vi "PID control.vi"() -> ()   [LabVIEW 2017]
uses:
  <vilib>/Simulation/Scripting/Companion Diagram/SimConfigNode/SimParams.ctl
  <vilib>/Simulation/Scripting/Companion Diagram/SimConfigNode/_simSolvers.ctl
  <vilib>/Simulation/Implementation/Shared/SIMSCR Execution Mode.ctl
  <vilib>/Simulation/Param Hierarchy/Typedefs/SIMPH Param Control Actions.ctl
  <vilib>/Simulation/Implementation/Shared/NILVSim_ParamChanged.vi
  <vilib>/Simulation/Implementation/Shared/NILVSIM_BeginStep.vi
  <vilib>/Simulation/Implementation/Shared/NILVSim_Manager.vi
  <vilib>/Utility/error.llb/Clear Errors.vi
  <vilib>/Simulation/Implementation/Shared/NILVSim_FinalizeModel.vi
  <vilib>/DAQmx/read.llb/DAQmx Read (Counter DBL 1Chan 1Samp).vi
  <vilib>/DAQmx/read.llb/DAQmx Read (Digital Bool 1Line 1Point).vi
  917b7e52-755f-4d44-bea8-9e7c9beac24e.vi
  a58f9967-76f1-4ebc-ad3d-26e75a3ca160.vi
  <vilib>/DAQmx/write.llb/DAQmx Write (Analog DBL 1Chan 1Samp).vi
  <vilib>/DAQmx/create/channels.llb/DAQmx Create Channel (AO-Voltage-Basic).vi
  <vilib>/DAQmx/create/channels.llb/DAQmx Create Channel (DI-Digital Input).vi
  <vilib>/DAQmx/create/channels.llb/DAQmx Create Channel (CI-Count Edges).vi
  <vilib>/Simulation/Implementation/Shared/SIM Unbundle Sim Info.vi
  <vilib>/Simulation/Implementation/Shared/NILVSim_Initialize.vi
  <vilib>/Simulation/Utility/Implementation/NILVSim Get Time and IsAcceptedStep.vi
  <vilib>/Simulation/Implementation/Shared/SIMSH Read Queue.vi
  <vilib>/Simulation/Implementation/Shared/NILVSim_GetModelError.vi
  <vilib>/Simulation/Implementation/Shared/SIM Bundle Sim Info.vi
  <vilib>/DAQmx/miscellaneous.llb/DAQmx Fill In Error Info.vi
  <vilib>/Simulation/Implementation/XNodeFramework/SimXNode/SimX.xnode
  <vilib>/Simulation/Model Libraries/PID/SIM PID (Parallel).vi
  <vilib>/Simulation/Model Libraries/PID/SIM PID.vi
  <vilib>/Simulation/Scripting/Companion Diagram/SimConfigNode/SimDog.xnode
  <vilib>/Simulation/Model Libraries/PID/SIM PID (Academic).vi
  <vilib>/Simulation/Implementation/Shared/NI_SIM_Implementation.lvlib
panel:
  out "x circle":bool
  out "y circle":bool
  out "Point circle is drawing":dbl
  out "false":bool
  in  "Radius 2":dbl
  out "No of Points":dbl
  out "Numeric y 2":dbl
  out "Y array 2":dbl[](array[numeric])
  out "array Y length 2":dbl
  out "Numeric x 2":dbl
  out "X array 2":dbl[](array[numeric])
  out "array x Length 2":dbl
  in  "stage circle":T1(ring)
  in  "check instruc":bool
  out "down 2":bool
  out "down":bool
  out "right":bool
  out "x entered":dbl
  out "y enetred":dbl
  out "greater -1 x":bool
  out "less 1 x":bool
  out "direction selected":dbl
  out "circle reset":bool
  in  "part circle":T2(ring)=enum."a"
  out "at 2f":bool
  out "Step 2J":bool
  out "Step 2H":bool
  out "Shape drawing steps":enum16{"corner", "1st switch", "reverse"}(ring)
  out "Step 2D":bool
  out "Step 2C":bool
  out "c":bool
  in  "height":dbl
  in  "length":dbl
  in  "part":T3(ring)=enum."a"
  out "Step 2A":bool
  out "Step 2B":bool
  in  "Has encoders been reset?":enum16{"don't reset", "reset"}(ring)
  out "x distance currently being travelled":dbl
  out "y distance currently being travelled":dbl
  out "error calced":dbl
  out "p1 dis 2":dbl
  out "p1 dis":dbl
  out "error y":dbl
  out "calc distance y":dbl
  out "calc distanc x":dbl
  out "error x":dbl
  out "reached y":bool
  out "reached x":bool
  out "Numeric":dbl
  in  "Draw rectangle":bool
  in  "Draw circle":bool
  out "In drawing mode":bool
  in  "Right-Down":bool
  in  "Left-Up":bool
  in  "Left-Down":bool
  in  "Right-Up":bool
  in  "right":bool
  in  "left":bool
  in  "motor 2":dbl(slide)=1.5 scale=-10.0..10.0
  in  "down":bool
  in  "up":bool
  in  "Y Length":dbl=30.0
  in  "X Length":dbl=30.0
  in  "Motor 2 encoder":tag="Dev1/ctr1"
  out "Pulses M2":dbl format="%.2f"
  in  "Motor 1 encoder":tag="Dev1/ctr0"
  out "Pulses M1":dbl format="%.2f"
  out "Right":bool
  out "Bottom":bool
  out "Left":bool
  out "Top":bool
  in  "Switch 4/Line 3":tag="Dev1/port0/line3"
  in  "Switch 3/Line 2":tag="Dev1/port0/line2"
  in  "Switch 2/Line 1":tag="Dev1/port0/line1"
  in  "Switch 1/Line 0":tag="Dev1/port0/line0"
  in  "Motor stop":bool
  in  "Motor 1":tag="Dev1/ao0"
  in  "max Voltage":dbl=10.0
  in  "Min Voltage":dbl=-10.0
  in  "Motor 2":tag="Dev1/ao1"
  in  "motor 1":dbl(slide)=1.5 scale=-10.0..10.0
  in  "stop":bool
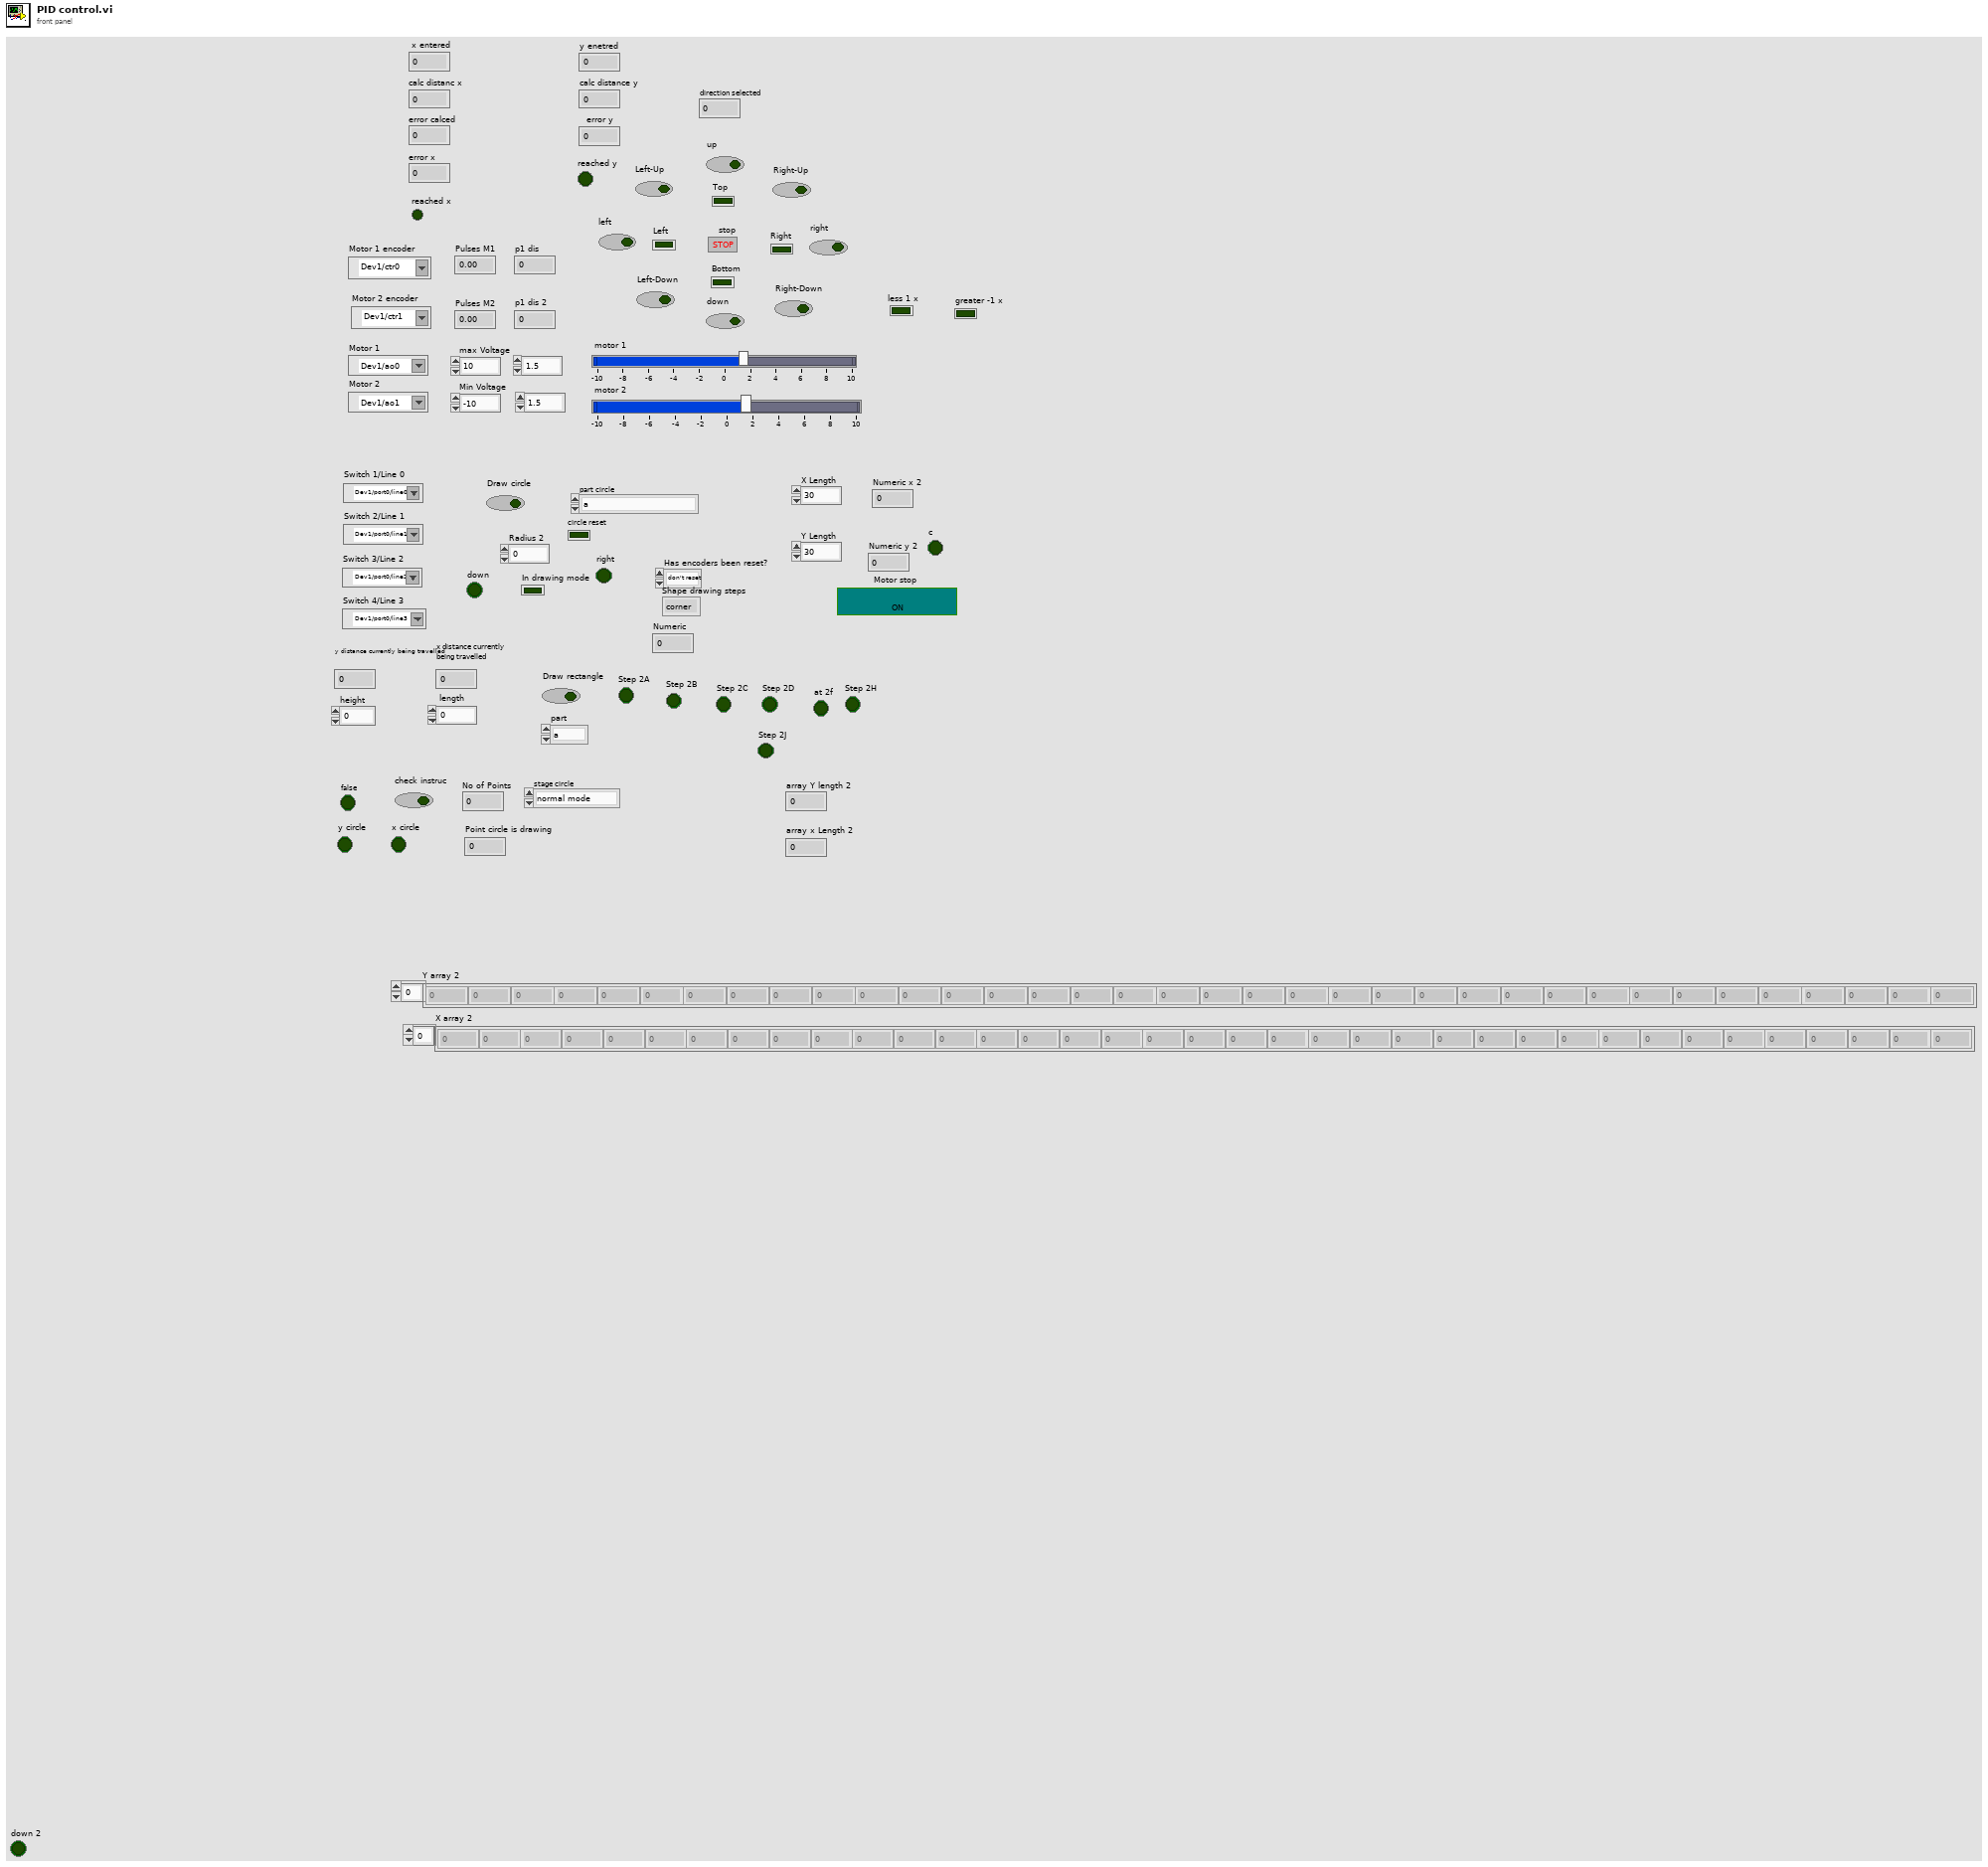
[diagram p1: front panel]
types:
  T1 = enum16{"normal mode", "create points", "draw points", "reset draw counter"}
  T2 = enum16{"nothing", "circle", "reset_before_circle", "radius_travel", "going right", "going down", "a"}
  T3 = enum16{"nothing", "j", "i", "h", "g", "f", "e", "d", "c", "b", "a"}
  T4 = enum16{"normal mode", "create points", "draw points"}
  T5 = enum16{"Simulate to Completion", "Single Time-Step Simulation (Fixed Step Only)"}
  T6 = typedef "SIMSCR Execution Mode.ctl" = enum16{"Simulate to Completion", "Single Time-Step Simulation (Fixed Step Only)"}
  T7 = typedef "SIMPH Param Control Actions.ctl" = enum16{"get params", "set params"}
  T8 = cluster{"SIMSH Sim Time":dbl, "SIM PID Derivative Gain.vi":cluster{"output":dbl}, "SIM PID Derivative Gain.vi - SIMSH":cluster{"SIMSH Sim Time":dbl, "t 3":dbl, "Select 2":cluster{"s? t:f":dbl}, "Equal?":cluster{"x = y?":bool}, "Or":cluster{"x .or. y?":bool}, "Equal To 0?":cluster{"x = 0?":bool}}, "High Frequency [s] (Tf)":dbl, "Gain":cluster{"output":dbl}, "Summation":cluster{"Result":dbl}, "Integral Gain - series.vi":cluster{"output":dbl}, "Integral Gain - series.vi - SIMSH":cluster{"SIMSH Sim Time":dbl, "Select 2":cluster{"s? t:f":dbl}, "integral in gain?":bool, "Integrator":cluster{"output y(t)":dbl}, "Gain 2":cluster{"output":dbl}, "Select":cluster{"s? t:f":dbl}, "Equal To 0?":cluster{"x = 0?":bool}, "Reciprocal":cluster{"1/x":dbl}}}
  T9 = typedef "SimParams.ctl" = cluster{"Initial Time (s)":dbl, "Final Time (s)":dbl, "Step Size (s)":dbl, "ODE Solver":T10, "Minimum Step Size (s)":dbl, "Maximum Step Size (s)":dbl, "Relative Tolerance":dbl, "Absolute Tolerance":dbl, "Software Timing":bool, "Initial Step Size (s)":dbl, "Automatic Fixed Step Size?":bool, "Automatic Discrete Step Size?":bool, "Discrete Step Size (s)":dbl, "Calculate using Time Step":bool, "Solver Wired?":bool, "Prev.Frm.Expected End":u64, "Prev.Frm.Actual End":u64, "Prev.Frm.Finished Late?":bool, "Prev.Iter.Expected End":u64, "Prev.Iter.Actual End":u64, "Prev.Iter.Finished Late?":bool, "Expected Iteration Start":u64, "Actual Iteration Start":u64, "Expected Frame Start":u64, "Actual Frame Start":u64, "Source Name":string, "Name":string, "Period":i64, "Deadline":i64, "Offset":i64, "Start":i64, "Priority":i32, "Timeout":i32, "Processor":i32, "Mode":enum32{"No Change", "Process missed periods, maintain original phase", "Discard missed periods, maintain original phase", "Process missed periods, ignore original phase", "Discard missed periods, ignore original phase"}, "Wakeup reason":enum32{"Normal", "Aborted", "Asynchronous wakeup", "Timing source error", "Timed loop error", "Timeout"}, "Error":errorcluster, "Source Type":string, "Secondary Source Type":string, "Global End Time":u64, "Global Start Time":u64, "Full Solver Reset":bool, "Execution Mode":T6, "Nan/Inf Check":bool, "Custom Solver Library":string, "Solver Is Variable":bool, "custom solver name":string, "Signal Collection Decimation":u32}
  T10 = typedef "_simSolvers.ctl" = enum16{"Runge-Kutta 1 (Euler)", "Runge-Kutta 2", "Runge-Kutta 3", "Runge-Kutta 4", "Runge-Kutta 23 (variable)", "Runge-Kutta 45 (variable)", "BDF (variable)", "Adams-Moulton (variable)", "Rosenbrock (variable)", "Discrete States Only", "SDIRK 4 (variable)", "Radau 5 (variable)", "Radau 9 (variable)", "Radau 13 (variable)", "Radau [Variable Order] (variable)", "Gear's Method (variable)", "Linearizer", "State Query", "Trim Eval", "Custom Solver"}
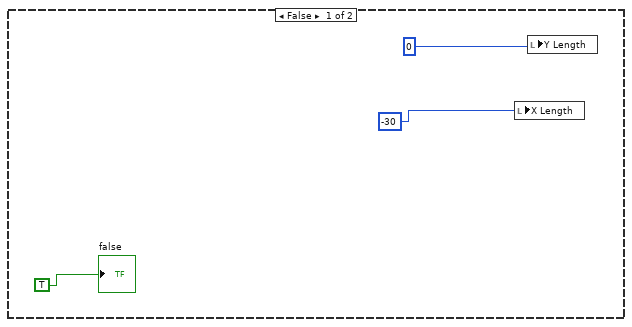
[diagram p2: hidden frame]
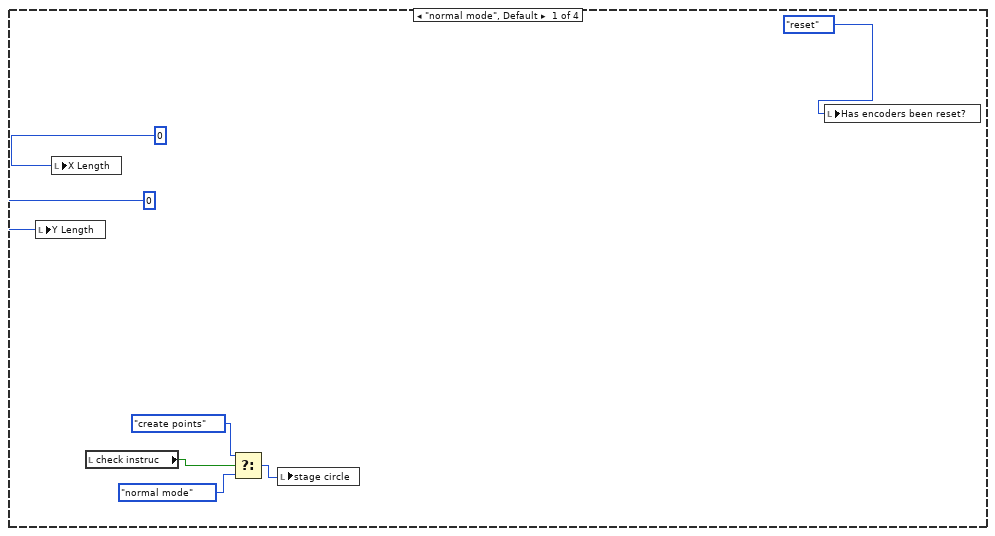
[diagram p3: hidden frame]
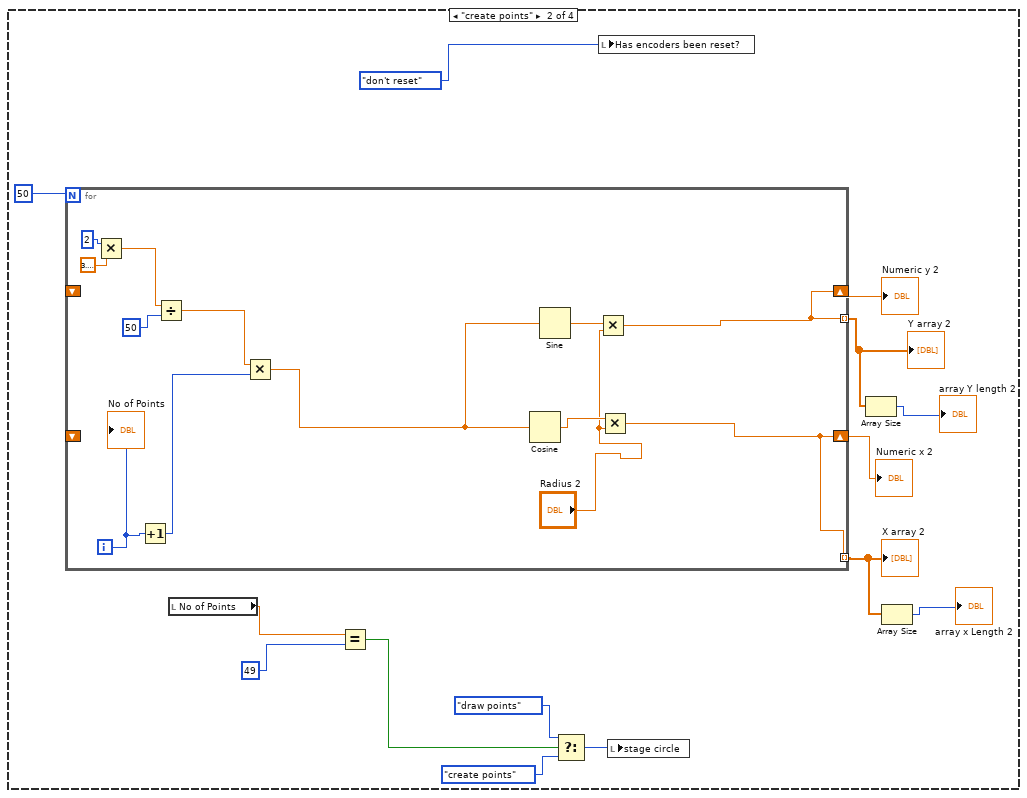
[diagram p4: hidden frame]
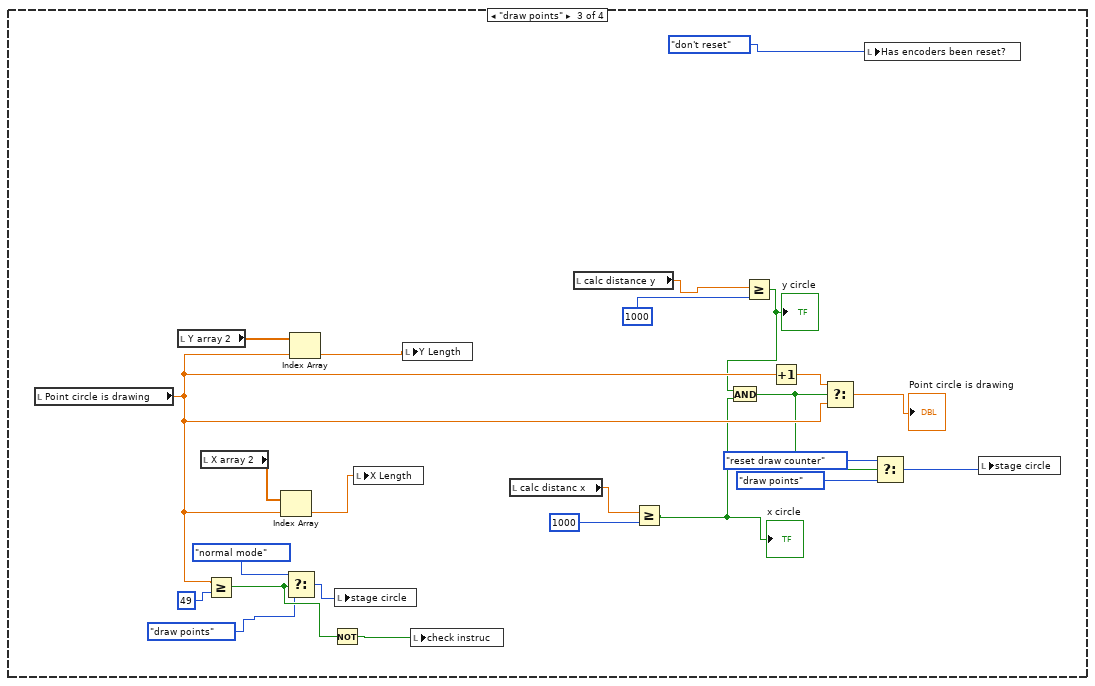
[diagram p5: hidden frame]
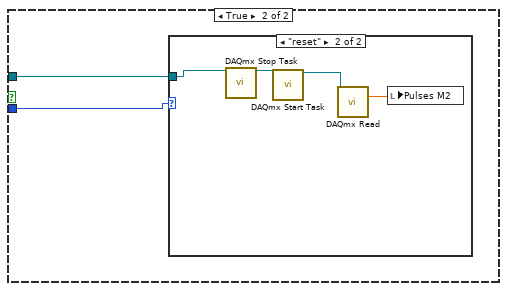
[diagram p6: hidden frame]
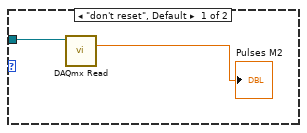
[diagram p7: hidden frame]
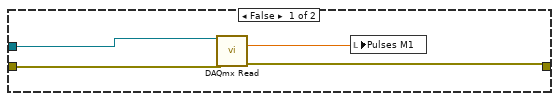
[diagram p8: hidden frame]
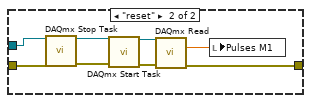
[diagram p9: hidden frame]
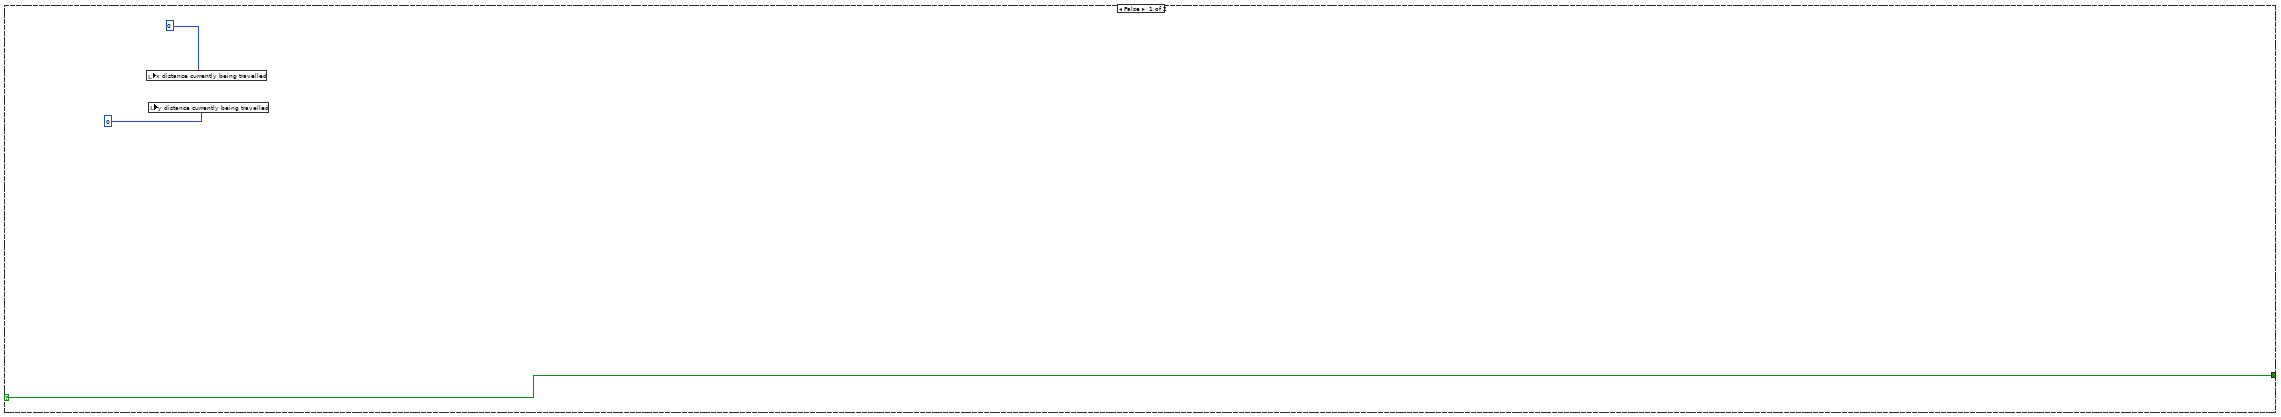
[diagram p10: hidden frame]
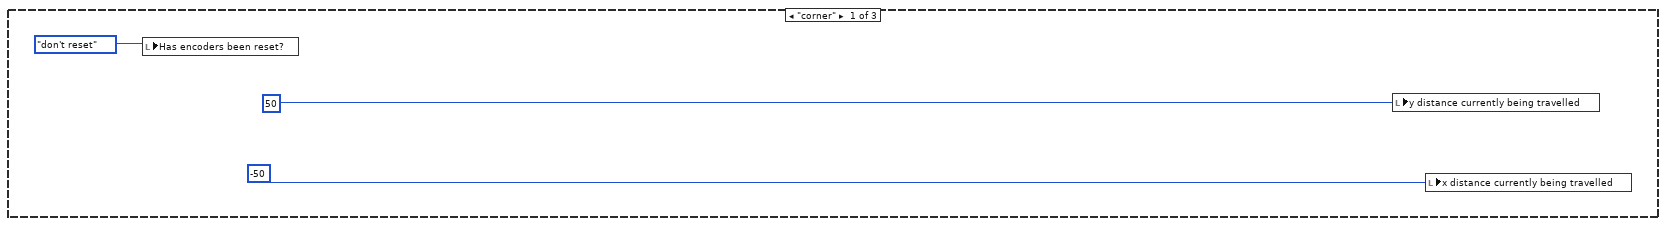
[diagram p11: hidden frame]
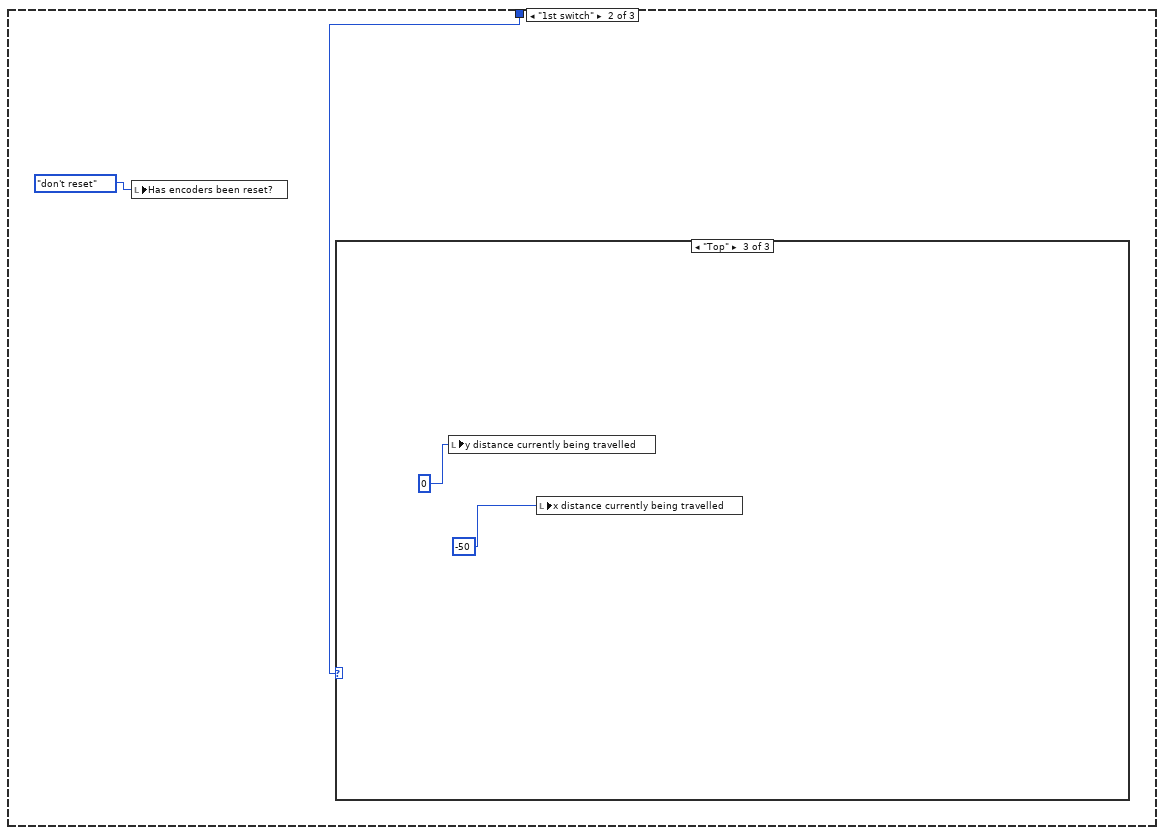
[diagram p12: hidden frame]
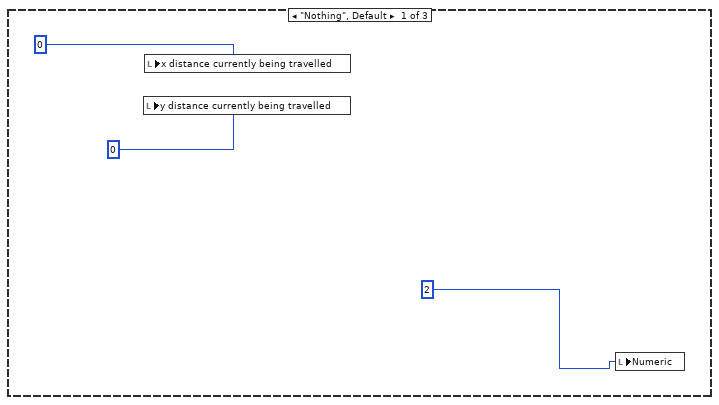
[diagram p13: hidden frame]
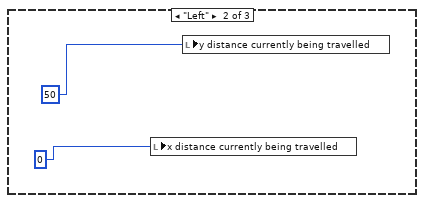
[diagram p14: hidden frame]
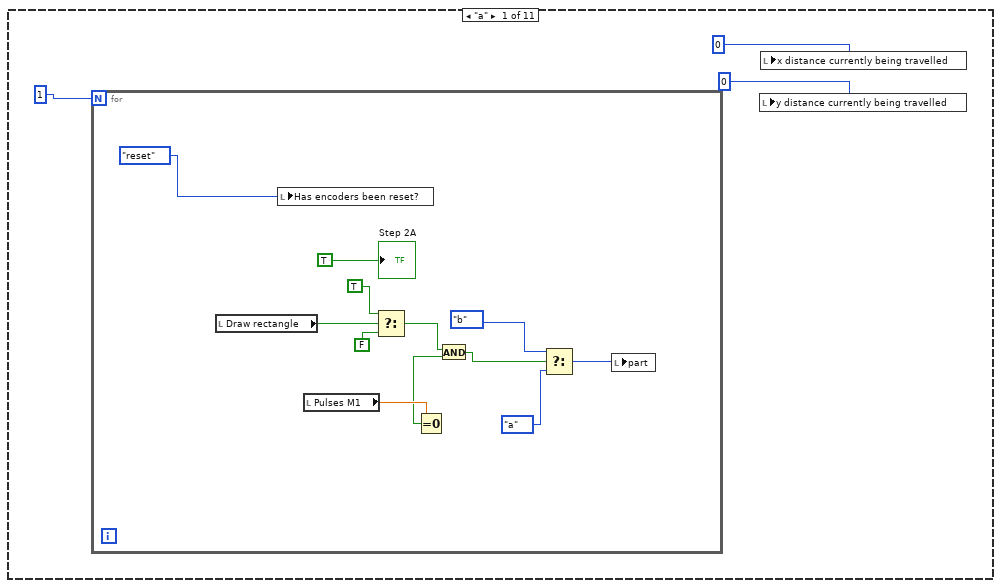
[diagram p15: hidden frame]
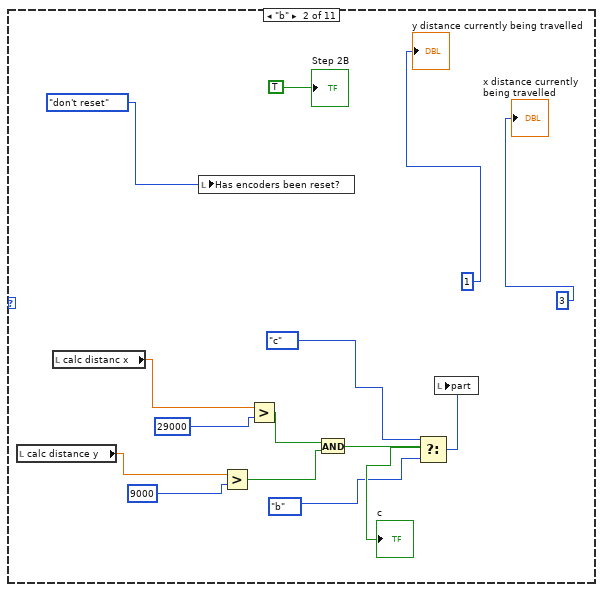
[diagram p16: hidden frame]
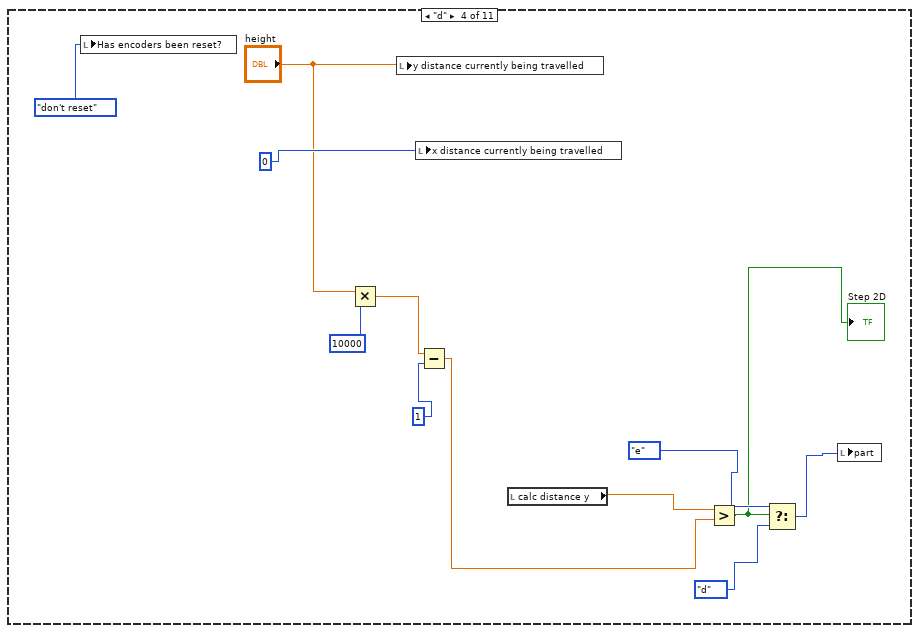
[diagram p17: hidden frame]
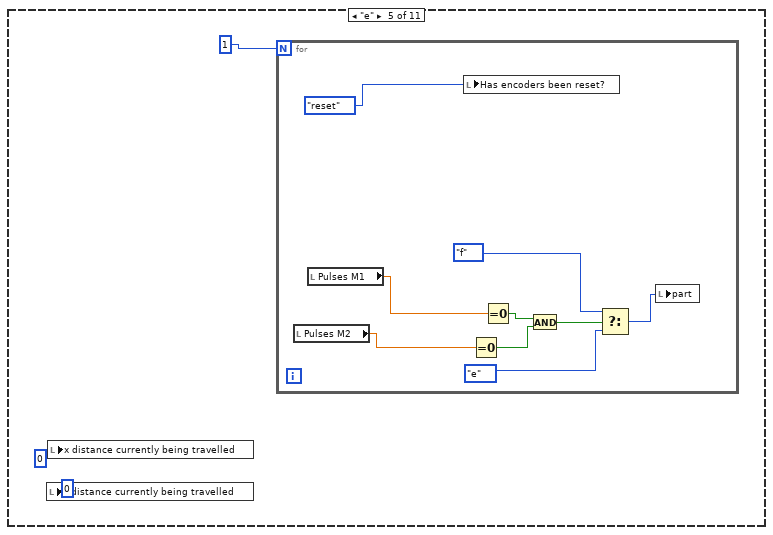
[diagram p18: hidden frame]
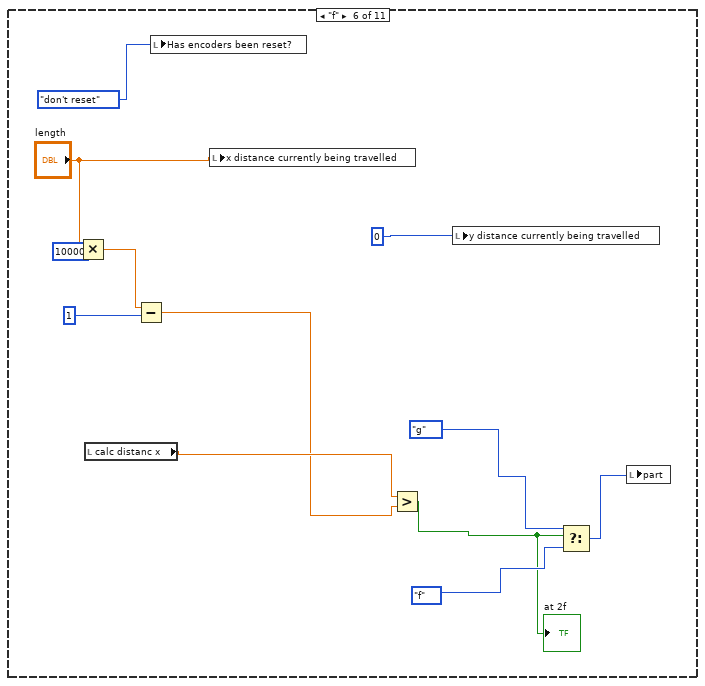
[diagram p19: hidden frame]
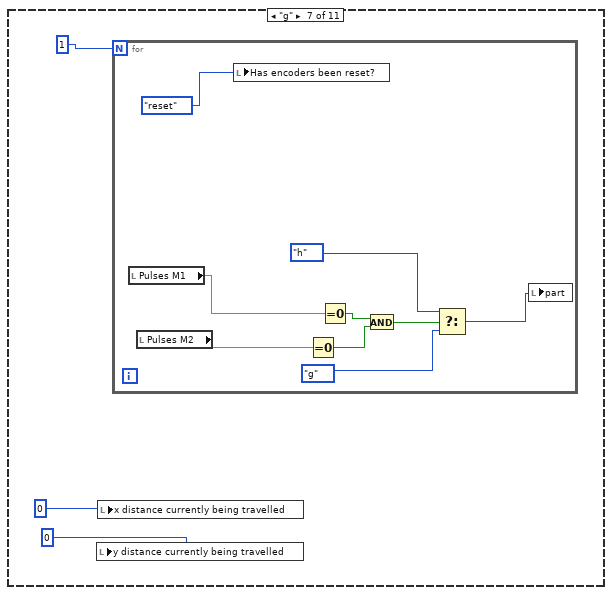
[diagram p20: hidden frame]
diagram:
  n1 = call-poly <vilib>:"DAQmx Create Virtual Channel.vi"("lines"="Switch 1/Line 0") -> ("task out"=w36:refnum<k21>, "error out"=w32:errorcluster)  [unwired: 13 in]
  n2 = call-poly <vilib>:"DAQmx Create Virtual Channel.vi"("lines"="Switch 2/Line 1") -> ("task out"=w35:refnum<k21>, "error out"=w31:errorcluster)  [unwired: 13 in]
  n3 = call-poly <vilib>:"DAQmx Create Virtual Channel.vi"("lines"="Switch 3/Line 2") -> ("task out"=w34:refnum<k21>, "error out"=w30:errorcluster)  [unwired: 13 in]
  n4 = call-poly <vilib>:"DAQmx Create Virtual Channel.vi"("lines"="Switch 4/Line 3") -> ("task out"=w33:refnum<k21>, "error out"=w29:errorcluster)  [unwired: 13 in]
  n5 = call <vilib>:"DAQmx Start Task.vi"("task/channels in"=w36, "error in"=w32) -> ("task out"=w28:refnum<k21>, "error out"=w26:errorcluster)  [unwired: 12 in]
  n6 = call <vilib>:"DAQmx Start Task.vi"("task/channels in"=w35, "error in"=w31) -> ("task out"=w24:refnum<k21>, "error out"=w21:errorcluster)  [unwired: 12 in]
  n7 = call <vilib>:"DAQmx Start Task.vi"("task/channels in"=w34, "error in"=w30) -> ("task out"=w23:refnum<k21>, "error out"=w20:errorcluster)  [unwired: 12 in]
  n8 = call <vilib>:"DAQmx Start Task.vi"("task/channels in"=w33, "error in"=w29) -> ("task out"=w22:refnum<k21>, "error out"=w19:errorcluster)  [unwired: 12 in]
  n9 = call-poly <vilib>:"DAQmx Create Virtual Channel.vi"("maximum value"="max Voltage", "minimum value"="Min Voltage", "physical channels"="Motor 1") -> ("task out"=w46:refnum<k21>, "error out"=w42:errorcluster)  [unwired: 11 in]
  n10 = call-poly <vilib>:"DAQmx Create Virtual Channel.vi"("counter"="Motor 2 encoder") -> ("task out"=w6:refnum<k21>)  [unwired: 13 in, 1 out]
  n11 = call-poly <vilib>:"DAQmx Create Virtual Channel.vi"("maximum value"="max Voltage", "minimum value"="Min Voltage", "physical channels"="Motor 2") -> ("task out"=w49:refnum<k21>, "error out"=w41:errorcluster)  [unwired: 11 in]
  n12 = call-poly <vilib>:"DAQmx Create Virtual Channel.vi"("counter"="Motor 1 encoder") -> ("task out"=w7:refnum<k21>, "error out"=w2:errorcluster)  [unwired: 13 in]
  n13 = call <vilib>:"DAQmx Start Task.vi"("task/channels in"=w6) -> ("task out"=w1:refnum<k21>)  [unwired: 13 in, 1 out]
  n14 = call <vilib>:"DAQmx Start Task.vi"("task/channels in"=w7) -> ("task out"=w3:refnum<k21>)  [unwired: 13 in, 1 out]
  n15 = while {
    tunnel: w49 -> [w231]
    tunnel: [w228] -> w48
    tunnel: w46 -> [w225]
    tunnel: [w224] -> w45
    tunnel: w42 -> [w222]
    tunnel: w41 -> [w221]
    tunnel: w28 -> [w215]
    tunnel: [w214] -> w27
    tunnel: w26 -> [w213]
    tunnel: [w212] -> w25
    tunnel: w24 -> [w211]
    tunnel: w23 -> [w210]
    tunnel: w22 -> [w209]
    tunnel: w21 -> [w208]
    tunnel: w20 -> [w207]
    tunnel: w19 -> [w206]
    tunnel: [w205] -> w18
    tunnel: [w204] -> w17
    tunnel: [w203] -> w16
    tunnel: [w202] -> w15
    tunnel: [w201] -> w14
    tunnel: [w200] -> w13
    tunnel: [w134] -> w10
    tunnel: w3 -> [w136]
    tunnel: w2 -> [w135]
    tunnel: w1 -> [w132]
    stop <- "stop" stop-if-true
    (unwired) TRUE
    n16 = Or(x="Draw circle", y="Draw rectangle") -> (x .or. y?=w144:bool)
    n17 = case shown="True" "check instruc" {
      frame False {
        n18 = local write "X Length"(-30) -> ()
        n19 = local write "Y Length"(0) -> ()
        "false" <- TRUE
      }
      frame True {
        n20 = case shown="\"reset draw counter\"" "stage circle" {
          frame "normal mode", Default {
            n21 = local write "Y Length"(0) -> ()
            n22 = local write "X Length"(0) -> ()
            n23 = local read "check instruc"() -> (w237:bool)
            n24 = Select(t=T4."create points", s=w237, f=T4."normal mode") -> (s? t:f=w238:T4)
            n25 = local write "stage circle"(w238) -> ()
            n26 = local write "Has encoders been reset?"(enum16{"don't reset", "reset"}."reset") -> ()
          }
          frame "create points" {
            n27 = for {
              N: 50 -> [_]
              shift-right: [w259] -> w250
              shift-left: _ -> [_]
              tunnel: [w259] -> w255 mode=indexing
              shift-right: [w258] -> w252
              shift-left: _ -> [_]
              tunnel: [w258] -> w254 mode=indexing
              i -> [w260]
              n28 = Multiply(x=2, y=3.141592653589793) -> (x*y=w263:dbl)
              n29 = Increment(x=w260) -> (x+1=w261:i32)
              n30 = Divide(x=w263, y=50) -> (x/y=w265:dbl)
              n31 = Multiply(x=w265, y=w261) -> (x*y=w262:dbl)
              n32 = Cosine(x=w262) -> (cos(x)=w268:dbl)
              n33 = Sine(x=w262) -> (sin(x)=w269:dbl)
              n34 = Multiply(x=w269, y="Radius 2") -> (x*y=w259:dbl)
              n35 = Multiply(x=w268, y="Radius 2") -> (x*y=w258:dbl)
              "No of Points" <- w260
            }
            "Numeric y 2" <- w250
            "Y array 2" <- w255
            "Numeric x 2" <- w252
            "X array 2" <- w254
            n36 = local read "No of Points"() -> (w249:dbl)
            n37 = Equal?(x=w249, y=49) -> (x = y?=w244:bool)
            n38 = Select(t=T4."draw points", s=w244, f=T4."create points") -> (s? t:f=w256:T4)
            n39 = local write "Has encoders been reset?"(enum16{"don't reset", "reset"}."don't reset") -> ()
            n40 = local write "stage circle"(w256) -> ()
            n41 = Array Size(array=w255) -> (size(s)=→"array Y length 2":i32)
            n42 = Array Size(array=w254) -> (size(s)=→"array x Length 2":i32)
          }
          frame "draw points" {
            n43 = local read "Point circle is drawing"() -> (w284:dbl)
            n44 = local read "Y array 2"() -> (w292:dbl[])
            n45 = local read "X array 2"() -> (w293:dbl[])
            n46 = Greater Or Equal?(x=w284, y=49) -> (x >= y?=w283:bool)
            n47 = Index Array(array=w293, index=w284) -> (element=w287:dbl)
            n48 = Select(t=T1."normal mode", s=w283, f=T1."draw points") -> (s? t:f=w288:T1)
            n49 = Index Array(array=w292, index=w284) -> (element=w286:dbl)
            n50 = Not(x=w283) -> (.not. x?=w282:bool)
            n51 = local write "stage circle"(w288) -> ()
            n52 = local write "X Length"(w287) -> ()
            n53 = local write "Y Length"(w286) -> ()
            n54 = local write "check instruc"(w282) -> ()
            n55 = local read "calc distanc x"() -> (w277:dbl)
            n56 = local read "calc distance y"() -> (w280:dbl)
            n57 = Greater Or Equal?(x=w277, y=1000) -> (x >= y?=w276:bool)
            "x circle" <- w276
            n58 = Greater Or Equal?(x=w280, y=1000) -> (x >= y?=w281:bool)
            "y circle" <- w281
            n59 = And(x=w281, y=w276) -> (x .and. y?=w275:bool)
            n60 = Increment(x=w284) -> (x+1=w291:dbl)
            n61 = Select(t=w291, s=w275, f=w284) -> (s? t:f=→"Point circle is drawing":dbl)
            n62 = local write "Has encoders been reset?"(enum16{"don't reset", "reset"}."don't reset") -> ()
            n63 = Select(t=T1."reset draw counter", s=w275, f=T1."draw points") -> (s? t:f=w274:T1)
            n64 = local write "stage circle"(w274) -> ()
          }
          frame "reset draw counter" {
            n65 = for {
              N: 1 -> [_]
              n66 = local read "Pulses M2"() -> (w302:dbl)
              n67 = local read "Pulses M1"() -> (w303:dbl)
              n68 = Equal To 0?(x=w302) -> (x = 0?=w300:bool)
              n69 = Equal To 0?(x=w303) -> (x = 0?=w299:bool)
              n70 = local write "Has encoders been reset?"(enum16{"don't reset", "reset"}."reset") -> ()
              n71 = And(x=w299, y=w300) -> (x .and. y?=w301:bool)
              n72 = Select(t=T1."draw points", s=w301, f=T1."reset draw counter") -> (s? t:f=w304:T1)
              n73 = local write "stage circle"(w304) -> ()
            }
            n74 = local write "X Length"(0) -> ()
            n75 = local write "Y Length"(0) -> ()
          }
        }
      }
    }
    n76 = local read "error y"() -> (w103:dbl)
    n77 = local read "error y"() -> (w102:dbl)
    n78 = local read "error x"() -> (w104:dbl)
    n79 = local read "error y"() -> (w118:dbl)
    n80 = local read "error y"() -> (w115:dbl)
    n81 = local read "error x"() -> (w111:dbl)
    n82 = local read "error x"() -> (w110:dbl)
    n83 = local read "error y"() -> (w119:dbl)
    n84 = local read "error x"() -> (w120:dbl)
    n85 = Less Than 0?(x=w103) -> (x < 0?=w101:bool)
    n86 = Less Than 0?(x=w104) -> (x < 0?=w100:bool)
    n87 = Greater Than 0?(x=w102) -> (x > 0?=w99:bool)
    n88 = Less Than 0?(x=w115) -> (x < 0?=w113:bool)
    n89 = Equal To 0?(x=w120) -> (x = 0?=w114:bool)
    n90 = Greater Than 0?(x=w118) -> (x > 0?=w117:bool)
    n91 = local read "error y"() -> (w96:dbl)
    n92 = local read "error x"() -> (w95:dbl)
    n93 = Greater Than 0?(x=w111) -> (x > 0?=w109:bool)
    n94 = Equal To 0?(x=w119) -> (x = 0?=w108:bool)
    n95 = Less Than 0?(x=w110) -> (x < 0?=w107:bool)
    n96 = And(x=w101, y=w100) -> (x .and. y?=w97:bool)
    n97 = And(x=w100, y=w99) -> (x .and. y?=w98:bool)
    n98 = And(x=w117, y=w114) -> (x .and. y?=w116:bool)
    n99 = And(x=w114, y=w113) -> (x .and. y?=w112:bool)
    n100 = local read "error y"() -> (w91:dbl)
    n101 = And(x=w109, y=w108) -> (x .and. y?=w106:bool)
    n102 = And(x=w108, y=w107) -> (x .and. y?=w105:bool)
    n103 = Greater Than 0?(x=w96) -> (x > 0?=w94:bool)
    n104 = Greater Than 0?(x=w95) -> (x > 0?=w92:bool)
    n105 = Less Than 0?(x=w91) -> (x < 0?=w90:bool)
    n106 = And(x=w94, y=w92) -> (x .and. y?=w93:bool)
    n107 = And(x=w92, y=w90) -> (x .and. y?=w89:bool)
    n108 = Select(t=1, s=w116, f=0) -> (s? t:f=w184:i32)
    n109 = Select(t=10, s=w105, f=0) -> (s? t:f=w182:i32)
    n110 = Select(t=2, s=w112, f=0) -> (s? t:f=w183:i32)
    n111 = Select(t=100, s=w93, f=0) -> (s? t:f=w180:i32)
    n112 = Select(t=200, s=w97, f=0) -> (s? t:f=w179:i32)
    n113 = Select(t=20, s=w106, f=0) -> (s? t:f=w181:i32)
    n114 = Select(t=1000, s=w98, f=0) -> (s? t:f=w178:i32)
    n115 = Select(t=2000, s=w89, f=0) -> (s? t:f=w164:i32)
    n116 = Add(x=w184, y=w183) -> (x+y=w177:i32)
    n117 = Add(x=w182, y=w181) -> (x+y=w176:i32)
    n118 = Add(x=w180, y=w179) -> (x+y=w175:i32)
    n119 = Add(x=w178, y=w164) -> (x+y=w163:i32)
    n120 = Add(x=w177, y=w176) -> (x+y=w174:i32)
    n121 = Add(x=w175, y=w163) -> (x+y=w162:i32)
    n122 = call-poly <vilib>:"DAQmx Read.vi"("task/channels in"=w215, "error in"=w213) -> ("task out"=w214:refnum<k21>, "data"=w146:bool, "error out"=w212:errorcluster)  [unwired: 11 in]
    "Top" <- w146
    n123 = call-poly <vilib>:"DAQmx Read.vi"("task/channels in"=w211, "error in"=w208) -> ("task out"=w205:refnum<k21>, "data"=w155:bool, "error out"=w202:errorcluster)  [unwired: 11 in]
    "Bottom" <- w155
    n124 = call-poly <vilib>:"DAQmx Read.vi"("task/channels in"=w210, "error in"=w207) -> ("task out"=w204:refnum<k21>, "data"=w154:bool, "error out"=w201:errorcluster)  [unwired: 11 in]
    "Right" <- w154
    n125 = call-poly <vilib>:"DAQmx Read.vi"("task/channels in"=w209, "error in"=w206) -> ("task out"=w203:refnum<k21>, "data"=w153:bool, "error out"=w200:errorcluster)  [unwired: 11 in]
    "Left" <- w153
    n126 = Add(x=w174, y=w162) -> (x+y=w88:i32)
    "direction selected" <- w88
    n127 = Multiply(x="Y Length", y=10) -> (x*y=w59:dbl)
    "y enetred" <- w59
    n128 = local read "Pulses M1"() -> (w133:dbl)
    n129 = local read "Pulses M2"() -> (w137:dbl)
    n130 = Divide(x=w133, y=52.56) -> (x/y=→"p1 dis":dbl)
    n131 = feedback #1() -> (w52:dbl)  [unwired: 1 in]
    "calc distance y" <- w52
    n132 = formula code="if (Ylength==0)\nYerror=0;\n else  \nif(Ylength<0)\nYerror= Ylength+calculating_y_dis;\nelse\nYerror= Ylength-calculating_y_dis;\n\nif (calculating_y_dis>1000)\nstay=0;\nif (stay==0 )\nYerror=0;"("Ylength"=w59, "calculating_y_dis"=w52, "stay"=1) -> ("Yerror"=w122:dbl)
    n133 = Divide(x=w137, y=52.56) -> (x/y=→"p1 dis 2":dbl)
    n134 = formula code="X=((PulseM1/52.56)+(PulseM2/52.56))/2.0;\nY=((PulseM1/52.56)+(PulseM2/52.56))/2.0;"("PulseM1"=w133, "PulseM2"=w137) -> ("X"=w56:dbl, "Y"=w57:dbl)
    n135 = Multiply(x=1000, y=w57) -> (x*y=w74:dbl)
    n136 = xnode "PID"("Error"=w122) -> ("Output"=w73:dbl)  [unwired: 2 in, 11 out]
    n137 = Multiply(x="X Length", y=10) -> (x*y=w62:dbl)
    "x entered" <- w62
    n138 = Multiply(x=1000, y=w56) -> (x*y=w69:dbl)
    n139 = Greater?(x=1, y=w73) -> (0:w86:bool)
    n140 = Less?(x=-1, y=w73) -> (x < y?=w84:bool)
    n141 = case shown="2000" w88 {
      tunnel: "motor 1" -> [w1040 w1043 w1046 w1053 w1057 w1061 w1067 w1073 w1079 w1084 w1091]
      tunnel: "motor 2" -> [w1037 w1045 w1048 w1051 w1056 w1059 w1065 w1071 w1077 w1085 w1090]
      tunnel: [w1036 w1045 w1047 w1050 w1056 w1058 w1064 w1070 w1076 w1082 w1089] -> w60
      tunnel: [w1039 w1042 w1046 w1052 w1057 w1060 w1066 w1072 w1078 w1083 w1088] -> w61
      frame 0, Default {
        n142 = Multiply(x=0, y=w1040) -> (x*y=w1039:dbl)
        n143 = Multiply(x=0, y=w1037) -> (x*y=w1036:dbl)
      }
      frame 1 {
        n144 = Multiply(x=-1, y=w1043) -> (x*y=w1042:dbl)
      }
      frame 2 {
        n145 = Multiply(x=-1.003, y=w1048) -> (x*y=w1047:dbl)
      }
      frame 10 {
        n146 = Multiply(x=-1, y=w1053) -> (x*y=w1052:dbl)
        n147 = Multiply(x=-1.1, y=w1051) -> (x*y=w1050:dbl)
      }
      frame 20 {
      }
      frame 100 {
        n148 = Multiply(x=0, y=w1061) -> (x*y=w1060:dbl)
        n149 = Multiply(x=1, y=w1059) -> (x*y=w1058:dbl)
      }
      frame 200 {
        n150 = Multiply(x=0, y=w1067) -> (x*y=w1066:dbl)
        n151 = Multiply(x=-1, y=w1065) -> (x*y=w1064:dbl)
      }
      frame 1000 {
        n152 = Multiply(x=-1, y=w1073) -> (x*y=w1072:dbl)
        n153 = Multiply(x=0, y=w1071) -> (x*y=w1070:dbl)
      }
      frame 2000 {
        n154 = Multiply(x=1, y=w1079) -> (x*y=w1078:dbl)
        n155 = Multiply(x=0, y=w1077) -> (x*y=w1076:dbl)
      }
      frame 4000 {
        n156 = Multiply(x=-1, y=w1084) -> (x*y=w1083:dbl)
        n157 = Multiply(x=0, y=w1085) -> (x*y=w1082:dbl)
      }
      frame 8000 {
        n158 = Multiply(x=-1, y=w1091) -> (x*y=w1088:dbl)
        n159 = Multiply(x=0, y=w1090) -> (x*y=w1089:dbl)
      }
    }
    n160 = And(x=w86, y=w84) -> (x .and. y?=w72:bool)
    "reached y" <- w72
    n161 = Select(t=w74, s=w72, f=w57) -> (s? t:f=w71:dbl)
    n162 = feedback-in #1(w71) -> ()
    n163 = Multiply(x=0, y=w73) -> (x*y=w82:dbl)
    n164 = Select(t=w82, s=w72, f=w73) -> (s? t:f=→"error y":dbl)
    n165 = local read "Numeric"() -> (w126:dbl)
    n166 = Or(x=w155, y=w154) -> (x .or. y?=w198:bool)
    n167 = local read "Draw circle"() -> (w130:bool)
    n168 = local read "Draw rectangle"() -> (w129:bool)
    n169 = And(x=w153, y=w146) -> (x .and. y?=w127:bool)
    n170 = Exclusive Or(1:w146, 2:w153) -> (0:w160:bool)
    n171 = Select(t=1, s=w153, f=0) -> (s? t:f=w145:i32)
    n172 = Select(t=2, s=w146, f=w145) -> (s? t:f=w150:i32)
    n173 = local read "Has encoders been reset?"() -> (w55:enum16{"don't reset", "reset"})
    n174 = Select(t=1, s=w160, f=w126) -> (s? t:f=w159:dbl)
    n175 = Select(t=2, s=w127, f=w159) -> (s? t:f=w157:dbl)
    n176 = feedback #2() -> (w67:bool)  [unwired: 1 in]
    "reached x" <- w67
    n177 = Select(t=w69, s=w67, f=w56) -> (s? t:f=w51:dbl)
    "calc distanc x" <- w51
    n178 = formula code="if (desired_xlength==0)\nXerror=0;\nelse\nif(desired_xlength>0)\nXerror=desired_xlength-actual_xLength;\nelse\nXerror=desired_xlength+actual_xLength;\n\nif (actual_xLength>1000)\nstay1=0;\nif (stay1==0)\nXerror=0;"("actual_xLength"=w51, "desired_xlength"=w62, "stay1"=1) -> ("Xerror"=w121:dbl)
    "error calced" <- w121
    n179 = xnode "PID 2"("Error"=w121) -> ("Output"=w77:dbl)  [unwired: 2 in, 11 out]
    n180 = Greater?(x=1, y=w77) -> (0:w65:bool)
    "greater -1 x" <- w65
    n181 = Less?(x=-1, y=w77) -> (x < y?=w66:bool)
    "less 1 x" <- w66
    n182 = And(x=w65, y=w66) -> (x .and. y?=w68:bool)
    n183 = Multiply(x=0, y=w77) -> (x*y=w79:dbl)
    n184 = feedback-in #2(w68) -> ()
    n185 = Or(x=w130, y=w129) -> (x .or. y?=w131:bool)
    n186 = Select(t=w79, s=w67, f=w77) -> (s? t:f=→"error x":dbl)
    n187 = call "Number To Enum.vim"("number"=w150, "enum type"=enum16{"Nothing", "Left", "Top"}."Nothing") -> ("number as enum"=w147:enum16{"Nothing", "Left", "Top"})
    n188 = case shown="True" w144 {
      selector: w144 -> [w832 w840]
      tunnel: [w832 w840] -> w161
      tunnel: w147 -> [_ w833]
      frame False {
        n189 = local write "x distance currently being travelled"(0) -> ()
        n190 = local write "y distance currently being travelled"(0) -> ()
      }
      frame True {
        n191 = local read "Numeric"() -> (w838:dbl)
        n192 = local read "Shape drawing steps"() -> (w835:enum16{"corner", "1st switch", "reverse"})
        n193 = Equal?(x=w838, y=2) -> (x = y?=w837:bool)
        n194 = Select(t=enum16{"corner", "1st switch", "reverse"}."reverse", s=w837, f=w835) -> (s? t:f=w834:enum16{"corner", "1st switch", "reverse"})
        n195 = case shown="\"reverse\"" w834 {
          tunnel: w833 -> [_ w844 _]
          frame "corner" {
            n196 = local write "Has encoders been reset?"(enum16{"don't reset", "reset"}."don't reset") -> ()
            n197 = local write "y distance currently being travelled"(50) -> ()
            n198 = local write "x distance currently being travelled"(-50) -> ()
          }
          frame "1st switch" {
            n199 = local write "Has encoders been reset?"(enum16{"don't reset", "reset"}."don't reset") -> ()
            n200 = case shown="\"Top\"" w844 {
              frame "Nothing", Default {
                n201 = local write "y distance currently being travelled"(0) -> ()
                n202 = local write "x distance currently being travelled"(0) -> ()
                n203 = local write "Numeric"(2) -> ()
              }
              frame "Left" {
                n204 = local write "x distance currently being travelled"(0) -> ()
                n205 = local write "y distance currently being travelled"(50) -> ()
              }
              frame "Top" {
                n206 = local write "y distance currently being travelled"(0) -> ()
                n207 = local write "x distance currently being travelled"(-50) -> ()
              }
            }
          }
          frame "reverse" {
            n208 = local read "Draw circle"() -> (w853:bool)
            n209 = case shown="False" w853 {
              tunnel: "part" -> [w856 _]
              frame False {
                n210 = case shown="\"c\"" w856 {
                  frame "a" {
                    n211 = for {
                      N: 1 -> [_]
                      n212 = local read "Draw rectangle"() -> (w860:bool)
                      n213 = local write "Has encoders been reset?"(enum16{"don't reset", "reset"}."reset") -> ()
                      n214 = local read "Pulses M1"() -> (w869:dbl)
                      n215 = Select(t=TRUE, s=w860, f=FALSE) -> (s? t:f=w863:bool)
                      n216 = Equal To 0?(x=w869) -> (x = 0?=w862:bool)
                      n217 = And(x=w863, y=w862) -> (x .and. y?=w861:bool)
                      n218 = Select(t=T3."b", s=w861, f=T3."a") -> (s? t:f=w868:T3)
                      n219 = local write "part"(w868) -> ()
                      "Step 2A" <- TRUE
                    }
                    n220 = local write "y distance currently being travelled"(0) -> ()
                    n221 = local write "x distance currently being travelled"(0) -> ()
                  }
                  frame "b" {
                    n222 = local read "calc distance y"() -> (w872:dbl)
                    n223 = local read "calc distanc x"() -> (w873:dbl)
                    n224 = local write "Has encoders been reset?"(enum16{"don't reset", "reset"}."don't reset") -> ()
                    n225 = Greater?(x=w872, y=9000) -> (0:w878:bool)
                    n226 = Greater?(x=w873, y=29000) -> (0:w877:bool)
                    n227 = And(x=w877, y=w878) -> (x .and. y?=w876:bool)
                    "c" <- w876
                    n228 = Select(t=T3."c", s=w876, f=T3."b") -> (s? t:f=w881:T3)
                    n229 = local write "part"(w881) -> ()
                    "x distance currently being travelled" <- 3
                    "y distance currently being travelled" <- 1
                    "Step 2B" <- TRUE
                  }
                  frame "c" {
                    n230 = for {
                      N: 1 -> [_]
                      n231 = local read "Pulses M1"() -> (w897:dbl)
                      n232 = local read "Pulses M2"() -> (w893:dbl)
                      n233 = local write "Has encoders been reset?"(enum16{"don't reset", "reset"}."reset") -> ()
                      n234 = Equal To 0?(x=w893) -> (x = 0?=w891:bool)
                      n235 = Equal To 0?(x=w897) -> (x = 0?=w892:bool)
                      n236 = And(x=w892, y=w891) -> (x .and. y?=w890:bool)
                      n237 = Select(t=T3."d", s=w890, f=T3."c") -> (s? t:f=w896:T3)
                      n238 = local write "part"(w896) -> ()
                    }
                    n239 = local write "y distance currently being travelled"(0) -> ()
                    n240 = local write "x distance currently being travelled"(0) -> ()
                    "Step 2C" <- TRUE
                  }
                  frame "d" {
                    n241 = local write "Has encoders been reset?"(enum16{"don't reset", "reset"}."don't reset") -> ()
                    n242 = Multiply(x="height", y=10000) -> (x*y=w906:dbl)
                    n243 = local write "y distance currently being travelled"("height") -> ()
                    n244 = local write "x distance currently being travelled"(0) -> ()
                    n245 = Subtract(x=w906, y=1) -> (x-y=w903:dbl)
                    n246 = local read "calc distance y"() -> (w908:dbl)
                    n247 = Greater?(x=w908, y=w903) -> (0:w899:bool)
                    "Step 2D" <- w899
                    n248 = Select(t=T3."e", s=w899, f=T3."d") -> (s? t:f=w909:T3)
                    n249 = local write "part"(w909) -> ()
                  }
                  frame "e" {
                    n250 = local write "y distance currently being travelled"(0) -> ()
                    n251 = local write "x distance currently being travelled"(0) -> ()
                    n252 = for {
                      N: 1 -> [_]
                      n253 = local read "Pulses M2"() -> (w915:dbl)
                      n254 = local read "Pulses M1"() -> (w916:dbl)
                      n255 = local write "Has encoders been reset?"(enum16{"don't reset", "reset"}."reset") -> ()
                      n256 = Equal To 0?(x=w915) -> (x = 0?=w921:bool)
                      n257 = Equal To 0?(x=w916) -> (x = 0?=w922:bool)
                      n258 = And(x=w922, y=w921) -> (x .and. y?=w920:bool)
                      n259 = Select(t=T3."f", s=w920, f=T3."e") -> (s? t:f=w914:T3)
                      n260 = local write "part"(w914) -> ()
                    }
                  }
                  frame "f" {
                    n261 = Multiply(x="length", y=10000) -> (x*y=w929:dbl)
                    n262 = local read "calc distanc x"() -> (w932:dbl)
                    n263 = Subtract(x=w929, y=1) -> (x-y=w926:dbl)
                    n264 = local write "Has encoders been reset?"(enum16{"don't reset", "reset"}."don't reset") -> ()
                    n265 = local write "x distance currently being travelled"("length") -> ()
                    n266 = Greater?(x=w932, y=w926) -> (0:w923:bool)
                    "at 2f" <- w923
                    n267 = local write "y distance currently being travelled"(0) -> ()
                    n268 = Select(t=T3."g", s=w923, f=T3."f") -> (s? t:f=w931:T3)
                    n269 = local write "part"(w931) -> ()
                  }
                  frame "g" {
                    n270 = local write "y distance currently being travelled"(0) -> ()
                    n271 = local write "x distance currently being travelled"(0) -> ()
                    n272 = for {
                      N: 1 -> [_]
                      n273 = local read "Pulses M1"() -> (w939:dbl)
                      n274 = local read "Pulses M2"() -> (w938:dbl)
                      n275 = local write "Has encoders been reset?"(enum16{"don't reset", "reset"}."reset") -> ()
                      n276 = Equal To 0?(x=w938) -> (x = 0?=w945:bool)
                      n277 = Equal To 0?(x=w939) -> (x = 0?=w946:bool)
                      n278 = And(x=w946, y=w945) -> (x .and. y?=w944:bool)
                      n279 = Select(t=T3."h", s=w944, f=T3."g") -> (s? t:f=w941:T3)
                      n280 = local write "part"(w941) -> ()
                    }
                  }
                  frame "h" {
                    n281 = local write "Has encoders been reset?"(enum16{"don't reset", "reset"}."don't reset") -> ()
                    n282 = local read "height"() -> (w950:dbl)
                    n283 = Multiply(x=w950, y=10000) -> (x*y=w958:dbl)
                    n284 = local write "y distance currently being travelled"(w950) -> ()
                    n285 = Subtract(x=w958, y=1) -> (x-y=w955:dbl)
                    n286 = local write "x distance currently being travelled"(0) -> ()
                    n287 = local read "calc distance y"() -> (w948:dbl)
                    n288 = Greater?(x=w948, y=w955) -> (0:w959:bool)
                    n289 = Select(t=T3."i", s=w959, f=T3."h") -> (s? t:f=w951:T3)
                    n290 = local write "part"(w951) -> ()
                    "Step 2H" <- TRUE
                  }
                  frame "i" {
                    n291 = for {
                      N: 1 -> [_]
                      n292 = local read "Pulses M1"() -> (w965:dbl)
                      n293 = local read "Pulses M2"() -> (w964:dbl)
                      n294 = local write "Has encoders been reset?"(enum16{"don't reset", "reset"}."reset") -> ()
                      n295 = Equal To 0?(x=w964) -> (x = 0?=w970:bool)
                      n296 = Equal To 0?(x=w965) -> (x = 0?=w971:bool)
                      n297 = And(x=w971, y=w970) -> (x .and. y?=w969:bool)
                      n298 = Select(t=T3."j", s=w969, f=T3."i") -> (s? t:f=w963:T3)
                      n299 = local write "part"(w963) -> ()
                    }
                    n300 = local write "y distance currently being travelled"(0) -> ()
                    n301 = local write "x distance currently being travelled"(0) -> ()
                  }
                  frame "j" {
                    (unwired) 1
                    n302 = local read "length"() -> (w975:dbl)
                    n303 = local read "calc distanc x"() -> (w977:dbl)
                    n304 = Multiply(x=w975, y=10000) -> (x*y=w972:dbl)
                    n305 = local write "Has encoders been reset?"(enum16{"don't reset", "reset"}."don't reset") -> ()
                    n306 = local write "x distance currently being travelled"(w975) -> ()
                    n307 = Greater?(x=w977, y=w972) -> (0:w980:bool)
                    n308 = local write "y distance currently being travelled"(0) -> ()
                    n309 = Select(t=T3."nothing", s=w980, f=T3."j") -> (s? t:f=w976:T3)
                    n310 = local write "part"(w976) -> ()
                    "Step 2J" <- TRUE
                  }
                  frame "nothing" {
                    n311 = local write "y distance currently being travelled"(0) -> ()
                    n312 = local write "x distance currently being travelled"(0) -> ()
                  }
                }
              }
              frame True {
                n313 = case shown="\"radius_travel\"" "part circle" {
                  frame "a" {
                    n314 = for {
                      N: 1 -> [_]
                      n315 = local read "Pulses M1"() -> (w994:dbl)
                      n316 = local read "Pulses M2"() -> (w993:dbl)
                      n317 = Equal To 0?(x=w994) -> (x = 0?=w996:bool)
                      n318 = Equal To 0?(x=w993) -> (x = 0?=w997:bool)
                      n319 = And(x=w996, y=w997) -> (x .and. y?=w995:bool)
                      "circle reset" <- w995
                      n320 = Select(t=T2."going right", s=w995, f=T2."a") -> (s? t:f=w991:T2)
                      n321 = local write "Has encoders been reset?"(enum16{"don't reset", "reset"}."reset") -> ()
                      n322 = local write "part circle"(w991) -> ()
                    }
                    n323 = local write "x distance currently being travelled"(0) -> ()
                    n324 = local write "y distance currently being travelled"(0) -> ()
                  }
                  frame "going down" {
                    n325 = local read "calc distance y"() -> (w1006:dbl)
                    n326 = Greater?(x=w1006, y=19000) -> (0:w1004:bool)
                    n327 = local write "Has encoders been reset?"(enum16{"don't reset", "reset"}."don't reset") -> ()
                    n328 = Select(t=T2."going right", s=w1004, f=T2."going down") -> (s? t:f=w1001:T2)
                    n329 = local write "y distance currently being travelled"(-2) -> ()
                    n330 = local write "x distance currently being travelled"(0) -> ()
                    n331 = local write "part circle"(w1001) -> ()
                    "down" <- TRUE
                  }
                  frame "going right" {
                    n332 = for {
                      N: 1 -> [_]
                      n333 = local read "Pulses M1"() -> (w1017:dbl)
                      n334 = local read "Pulses M2"() -> (w1016:dbl)
                      n335 = Equal To 0?(x=w1017) -> (x = 0?=w1019:bool)
                      n336 = Equal To 0?(x=w1016) -> (x = 0?=w1020:bool)
                      n337 = And(x=w1019, y=w1020) -> (x .and. y?=w1018:bool)
                      n338 = Select(t=T2."radius_travel", s=w1018, f=T2."going right") -> (s? t:f=w1014:T2)
                      n339 = local write "Has encoders been reset?"(enum16{"don't reset", "reset"}."reset") -> ()
                      n340 = local write "part circle"(w1014) -> ()
                    }
                    n341 = local write "x distance currently being travelled"(0) -> ()
                    n342 = local write "y distance currently being travelled"(0) -> ()
                    "right" <- TRUE
                  }
                  frame "radius_travel" {
                    n343 = local read "calc distanc x"() -> (w1023:dbl)
                    n344 = local write "x distance currently being travelled"(-4) -> ()
                    n345 = Greater?(x=w1023, y=39000) -> (0:w1027:bool)
                    n346 = local write "Has encoders been reset?"(enum16{"don't reset", "reset"}."don't reset") -> ()
                    n347 = Select(t=T2."going right", s=w1027, f=T2."going down") -> (s? t:f=w1022:T2)
                    n348 = local write "part circle"(w1022) -> ()
                    "down 2" <- TRUE
                  }
                  frame "reset_before_circle" {
                    n349 = local write "x distance currently being travelled"(0) -> ()
                    n350 = local write "y distance currently being travelled"(0) -> ()
                  }
                  frame "circle" {
                    n351 = local write "x distance currently being travelled"(0) -> ()
                    n352 = local write "y distance currently being travelled"(0) -> ()
                  }
                  frame "nothing" {
                    n353 = local write "x distance currently being travelled"(0) -> ()
                    n354 = local write "y distance currently being travelled"(0) -> ()
                  }
                }
              }
            }
            "Numeric" <- 2
          }
        }
      }
    }
    "In drawing mode" <- w161
    n355 = case shown="True" w131 {
      tunnel: w136 -> [w318 w323]
      tunnel: w135 -> [w319 w322]
      tunnel: [w316 w321] -> w134
      frame False {
        n356 = call-poly <vilib>:"DAQmx Read.vi"("task/channels in"=w318, "error in"=w319) -> ("data"=w317:dbl, "error out"=w316:errorcluster)  [unwired: 11 in, 1 out]
        n357 = local write "Pulses M1"(w317) -> ()
      }
      frame True {
        n358 = case shown="\"don't reset\", Default" "Has encoders been reset?" {
          tunnel: w323 -> [w327 w334]
          tunnel: w322 -> [w326 w333]
          tunnel: [w324 w335] -> w321
          frame "don't reset", Default {
            n359 = call-poly <vilib>:"DAQmx Read.vi"("task/channels in"=w327, "error in"=w326) -> ("data"=→"Pulses M1":dbl, "error out"=w324:errorcluster)  [unwired: 11 in, 1 out]
          }
          frame "reset" {
            n360 = call <vilib>:"DAQmx Stop Task.vi"("task/channels in"=w334, "error in"=w333) -> ("task out"=w332:refnum<k21>, "error out"=w331:errorcluster)  [unwired: 12 in]
            n361 = call <vilib>:"DAQmx Start Task.vi"("task/channels in"=w332, "error in"=w331) -> ("task out"=w330:refnum<k21>, "error out"=w329:errorcluster)  [unwired: 12 in]
            n362 = call-poly <vilib>:"DAQmx Read.vi"("task/channels in"=w330, "error in"=w329) -> ("data"=w328:dbl, "error out"=w335:errorcluster)  [unwired: 11 in, 1 out]
            n363 = local write "Pulses M1"(w328) -> ()
          }
        }
      }
    }
    n364 = And(x=w72, y=w67) -> (x .and. y?=w143:bool)
    n365 = Or(x=w198, y=w143) -> (x .or. y?=w197:bool)
    n366 = Or(x=w197, y="Motor stop") -> (x .or. y?=w199:bool)
    n367 = Or(x=w199, y="stop") -> (x .or. y?=w219:bool)
    n368 = Select(t=0.0, s=w219, f=w60) -> (s? t:f=w216:dbl)
    n369 = call-poly <vilib>:"DAQmx Write.vi"("task/channels in"=w225, "data"=w216, "error in"=w222) -> ("task out"=w226:refnum<k21>, "error out"=w227:errorcluster)  [unwired: 10 in, 1 out]
    n370 = Select(t=0.0 ("s? t:f"), s=w219, f=w61) -> (s? t:f=w217:dbl)
    n371 = call-poly <vilib>:"DAQmx Write.vi"("task/channels in"=w231, "data"=w217, "error in"=w221) -> ("task out"=w230:refnum<k21>, "error out"=w229:errorcluster)  [unwired: 10 in, 1 out]
    n372 = call <vilib>:"DAQmx Wait Until Done.vi"("task/channels in"=w230, "error in"=w229) -> ("error out"=w228:errorcluster)  [unwired: 12 in, 1 out]
    n373 = call <vilib>:"DAQmx Wait Until Done.vi"("task/channels in"=w226, "error in"=w227) -> ("error out"=w224:errorcluster)  [unwired: 12 in, 1 out]
    n374 = case shown="False" w131 {
      tunnel: w132 -> [w307 w309]
      tunnel: w55 -> [_ w308]
      frame False {
        n375 = call-poly <vilib>:"DAQmx Read.vi"("task/channels in"=w307) -> ("data"=w306:dbl)  [unwired: 12 in, 2 out]
        n376 = local write "Pulses M2"(w306) -> ()
      }
      frame True {
        n377 = case shown="\"reset\"" w308 {
          tunnel: w309 -> [w311 w314]
          frame "don't reset", Default {
            n378 = call-poly <vilib>:"DAQmx Read.vi"("task/channels in"=w311) -> ("data"=→"Pulses M2":dbl)  [unwired: 12 in, 2 out]
          }
          frame "reset" {
            n379 = call <vilib>:"DAQmx Stop Task.vi"("task/channels in"=w314) -> ("task out"=w313:refnum<k21>)  [unwired: 13 in, 1 out]
            n380 = call <vilib>:"DAQmx Start Task.vi"("task/channels in"=w313) -> ("task out"=w315:refnum<k21>)  [unwired: 13 in, 1 out]
            n381 = call-poly <vilib>:"DAQmx Read.vi"("task/channels in"=w315) -> ("data"=w312:dbl)  [unwired: 12 in, 2 out]
            n382 = local write "Pulses M2"(w312) -> ()
          }
        }
      }
    }
    n383 = call "Number To Enum.vim"("number"=w157, "enum type"=enum16{"corner", "1st switch", "reverse"}."corner") -> ("number as enum"=→"Shape drawing steps":enum16{"corner", "1st switch", "reverse"})
  }
  n384 = invoke on="motor 1" class="Slide (strict)" method="Reinit To Default"() -> ()  [unwired: 3 in, 3 out]
  n385 = call <vilib>:"Simple Error Handler.vi"("error source (\" \")"="you messed up" ("error source (\" \")"), "error in (no error)"=w48) -> ()  [unwired: 3 in, 5 out]
  n386 = call <vilib>:"Simple Error Handler.vi"("error source (\" \")"="you messed up" ("error source (\" \")"), "error in (no error)"=w45) -> ()  [unwired: 3 in, 5 out]
  n387 = call <vilib>:"DAQmx Clear Task.vi"("task in"=w27, "error in"=w25) -> ()  [unwired: 13 in, 1 out]
  n388 = call <vilib>:"DAQmx Clear Task.vi"("task in"=w17, "error in"=w14) -> ()  [unwired: 13 in, 1 out]
  n389 = call <vilib>:"DAQmx Clear Task.vi"("task in"=w18, "error in"=w15) -> ("error out"=w12:errorcluster)  [unwired: 13 in]
  n390 = call <vilib>:"DAQmx Clear Task.vi"("task in"=w16, "error in"=w13) -> ()  [unwired: 13 in, 1 out]
  n391 = call <vilib>:"Simple Error Handler.vi"("error in (no error)"=w12) -> ()  [unwired: 4 in, 5 out]
  n392 = call <vilib>:"Simple Error Handler.vi"("error source (\" \")"="you messed up" ("error source (\" \")"), "error in (no error)"=w10) -> ()  [unwired: 3 in, 5 out]
